vi "Router - Configure.vi"(8 "error in (no error)":errorcluster, 10 "Configuration Properties In":T1) -> (0 "error out":errorcluster, 2 "Configuration Properties Out":T1, 3 "Router Data Out":T4)   [LabVIEW 2016, in "PXImc Custom Device Engine.lvlib" / "PXImc Router.lvlib"]
uses:
  PXImc Router.lvlib
  Controls/Router Data.ctl
  Controls/Reader Data.ctl
  Controls/Table Index-Size.ctl
  Controls/Writer Data.ctl
  Controls/Router - Configuration.ctl
  Controls/Node Properties.ctl
  <vilib>/pximc/Initialize Writer Session (DBL).vi
  <vilib>/pximc/Initialize Reader Session (DBL).vi
  <vilib>/pximc/nipximc.lvlib
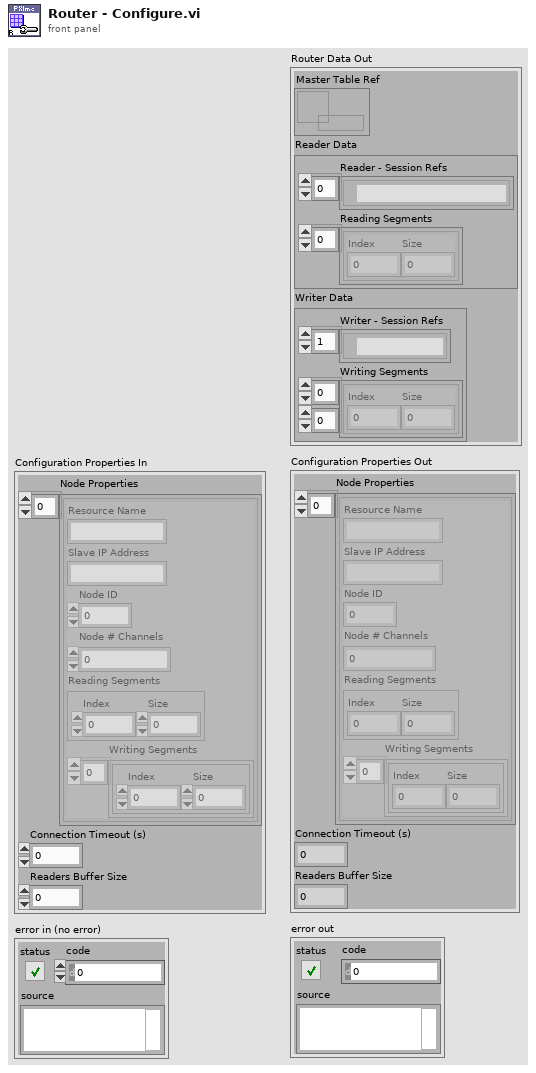
[diagram p1: front panel]
types:
  T1 = typedef "PXImc Custom Device Engine.lvlib/PXImc Router.lvlib/Router - Configuration.ctl" = cluster{"Node Properties":T2[], "Connection Timeout (s)":dbl, "Readers Buffer Size":u32}
  T2 = typedef "PXImc Custom Device Engine.lvlib/PXImc Router.lvlib/Node Properties.ctl" = cluster{"Resource Name":string, "Slave IP Address":string, "Node ID":u16, "Node # Channels":u32, "Reading Segments":T3, "Writing Segments":T3[]}
  T3 = typedef "PXImc Custom Device Engine.lvlib/PXImc Router.lvlib/Table Index-Size.ctl" = cluster{"Index":u32, "Size":u32}
  T4 = typedef "PXImc Custom Device Engine.lvlib/PXImc Router.lvlib/Router Data.ctl" = cluster{"Master Table Ref":refnum<data-value>, "Reader Data":T5, "Writer Data":T6}
  T5 = typedef "PXImc Custom Device Engine.lvlib/PXImc Router.lvlib/Reader Data.ctl" = cluster{"Reader - Session Refs":refnum<k21>[], "Reading Segments":T3[]}
  T6 = typedef "PXImc Custom Device Engine.lvlib/PXImc Router.lvlib/Writer Data.ctl" = cluster{"Writer - Session Refs":refnum<k21>[], "Writing Segments":T3[][]}
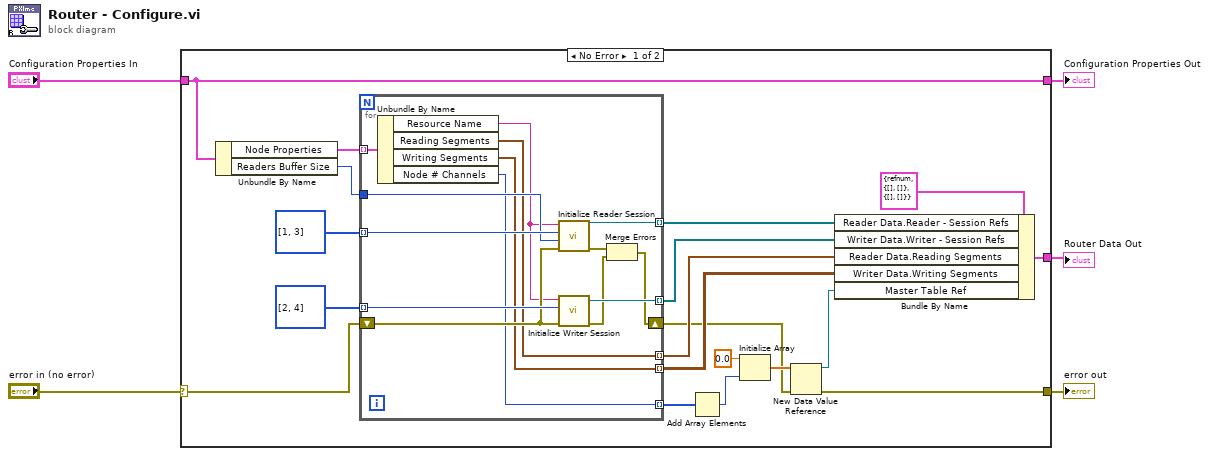
[diagram p0: block diagram]
diagram:
  n1 = case shown="No Error" "error in (no error)" {
    selector: "error in (no error)" -> [w13 w40]
    tunnel: [w24 _] -> w5
    tunnel: [w21 w40] -> w4
    tunnel: "Configuration Properties In" -> [w6 w39]
    tunnel: [w6 w39] -> w1
    frame No Error {
      n2 = Unbundle By Name(w6) -> ("Node Properties"=w14:T2[], "Readers Buffer Size"=w15:u32)
      n3 = for {
        tunnel: i32[] [1, 3] -> [w38] mode=indexing
        tunnel: i32[] [2, 4] -> [w37] mode=indexing
        tunnel: w15 -> [w36]
        tunnel: w14 -> [w35] mode=indexing
        tunnel: [w33] -> w12 mode=indexing
        tunnel: [w32] -> w11 mode=indexing
        tunnel: [w31] -> w10 mode=indexing
        tunnel: [w29] -> w9 mode=indexing
        tunnel: [w28] -> w8 mode=indexing
        shift-right: [w25] -> w7
        shift-left: w13 -> [w34]
        n4 = Unbundle By Name(w35) -> ("Resource Name"=w30:string, "Reading Segments"=w32:T3, "Writing Segments"=w31:T3[], "Node # Channels"=w33:u32)
        n5 = call-poly <vilib>:"Initialize Reader Session.vi"("error in (no error)"=w34, "buffer size"=w36, "writer's connection id (1)"=w38, "interface"=w30) -> ("error out"=w27:errorcluster, "session out"=w29:refnum<k21>)  [unwired: 6 in]
        n6 = call-poly <vilib>:"Initialize Writer Session.vi"("error in (no error)"=w34, "connection id (1)"=w37, "interface"=w30) -> ("error out"=w26:errorcluster, "session out"=w28:refnum<k21>)  [unwired: 7 in]
        n7 = Merge Errors(w27, w26) -> (w25:errorcluster)
      }
      n8 = Add Array Elements(numeric array=w12) -> (sum=w20:u32)
      n9 = Initialize Array(0.0 ("element"), w20) -> (w18:dbl[])
      n10 = New Data Value Reference(data value=w18, error in=w7) -> (data value reference=w23:refnum<data-value>, error out=w21:errorcluster)
      n11 = Bundle By Name(cluster=T4 {"Master Table Ref"=refnum, "Reader Data"={"Reader - Session Refs"=[], "Reading Segments"=[]}, "Writer Data"={"Writer - Session Refs"=[], "Writing Segments"=[]}} ("Cluster"), "Reader Data.Reader - Session Refs"=w9, "Writer Data.Writer - Session Refs"=w8, "Reader Data.Reading Segments"=w11, "Writer Data.Writing Segments"=w10, "Master Table Ref"=w23) -> (w24:T4)
    }
    frame Error {
    }
  }
  "Router Data Out" <- w5
  "error out" <- w4
  "Configuration Properties Out" <- w1
